vi "Create Self Enqueuer.vi"(6 "Name":string, 8 "error in":errorcluster, 10 "VI Refnum":refnum<vi>) -> (0 "error out":errorcluster, 3 "QDMH out":refnum<class "QDMH.lvclass">)   [LabVIEW 2023, in "QDMH.lvlib" / "QDMH.lvclass"]
doc: "This defines the unique name of the message queue spawned. It is required if a VI reference is not passed into this VI.\n\nThis defines the program named queue handle. If the caller VI passes its reference to this VI, the queue will take on the name of the caller VI. \n\n**Caution** using the caller VI name will not generate unique queue handles so it should only be used for top level applications that are not spawned as multiple instances."
uses:
  QDMH.lvclass
  Custom Controls/QDMH Message.ctl
  QDMH.lvclass/QDMH.ctl
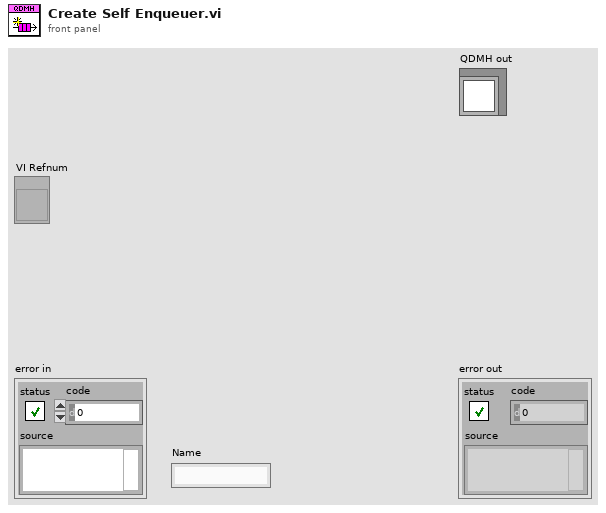
[diagram p1: front panel]
types:
  T1 = typedef "QDMH.lvlib/QDMH.lvclass/QDMH Message.ctl" = cluster{"State":string, "Data":variant}
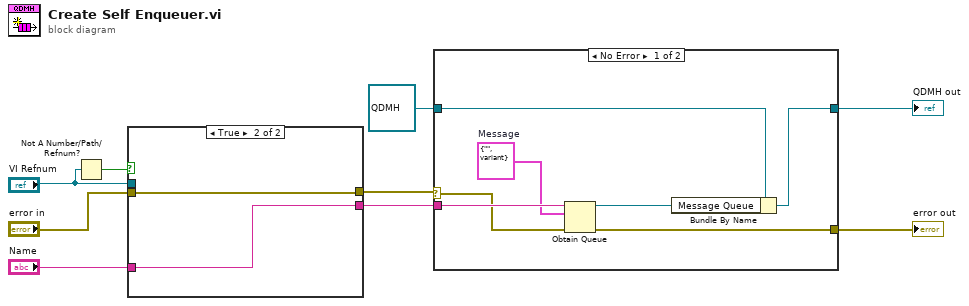
[diagram p0: block diagram]
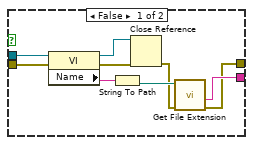
[diagram p2: hidden frame]
diagram:
  n1 = Not A Number/Path/Refnum?(number/path/refnum="VI Refnum") -> (NaN/Path/Refnum?=w2:bool)
  n2 = case shown="True" w2 {
    tunnel: "error in" -> [w18 w20]
    tunnel: [w12 w19] -> w5
    tunnel: [w10 w20] -> w4
    tunnel: "VI Refnum" -> [w15 _]
    tunnel: "Name" -> [_ w19]
    frame False {
      n3 = property class="VI"(reference=w15, error in=w18) -> (reference out=w16:refnum<vi>, error out=w17:errorcluster, "Name"=w14:string)
      n4 = String To Path(string=w14) -> (path=w13:path)
      n5 = Close Reference(reference=w16, error in (no error)=w17) -> (error out=w11:errorcluster)
      n6 = call <vilib>:"Get File Extension.vi"("error in (no error)"=w11, "file"=w13) -> ("error out"=w10:errorcluster, "filename without extension"=w12:string)  [unwired: 5 in, 3 out]
    }
    frame True {
    }
  }
  n7 = case shown="No Error" w4 {
    selector: w4 -> [w25 w29]
    tunnel: [w22 w29] -> w9
    tunnel: [w23 w28] -> w7
    tunnel: refnum<class "QDMH.lvclass"> refnum ("QDMH in") -> [w27 w28]
    tunnel: w5 -> [w26 _]
    frame No Error {
      w24 = T1 {"State"="", "Data"=variant}  # Message
      n8 = Obtain Queue(name (unnamed)=w26, element data type=w24, error in (no error)=w25) -> (queue out=w21:refnum<queue>, error out=w22:errorcluster)  [unwired: 2 in, 1 out]
      n9 = Bundle By Name(cluster=w27, "Message Queue"=w21) -> (w23:refnum<class "QDMH.lvclass">)
    }
    frame Error {
    }
  }
  "error out" <- w9
  "QDMH out" <- w7
